vi "Instrument Meas CCDF (LTE).vi"(6 "Count(Kpt)":i32(ring) items=["0"=0, "1"=1, "10"=10, "100"=100, "1000"=1000, "10000"=10000], 7 "OPC?(T)":bool=TRUE, 8 "error in":errorcluster {"code" format="%.0x"}, 10 "Timeout":u32=10000, 11 "Session In":refnum<visa-resource-name>="GPIB0::18::INSTR") -> (0 "error out":errorcluster {"code" format="%.0x"}, 1 "Formatted Data":dbl[](array[numeric]), 2 "Data(str)":string[](array[string]), 3 "Session Out":refnum<visa-resource-name>)   [LabVIEW 2018]
doc: "Launches the Instrument I/O Assistant, which you can use to communicate with message-based instruments and graphically parse the response. For example you can communicate with an instrument that uses a serial, Ethernet, or GPIB interface."
panel:
  # "Returns 10 scalar results:\n0. Average input power (in dBm)\n1. Probability at the average input power level (in %)\n2. Power level that has 10% of the power\n3. Power level that has 1% of the power\n4. Power level that has 0.1% of the power\n5. Power level that has 0.01% of the power\n6. Power level that has 0.001% of the power\n7. Power level that has 0.0001% of the power\n8. Peak power (in dB)\n9.Count"
  # "Returns 10 scalar results:\n0. Average input power (in dBm)\n1. Peak  (in dB)\n2. Pk @ (dBm)"
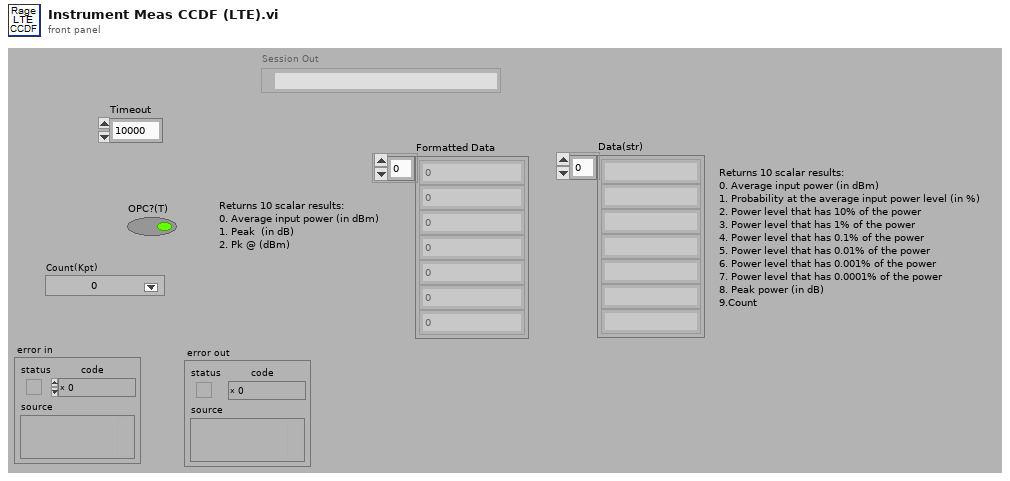
[diagram p1: front panel]
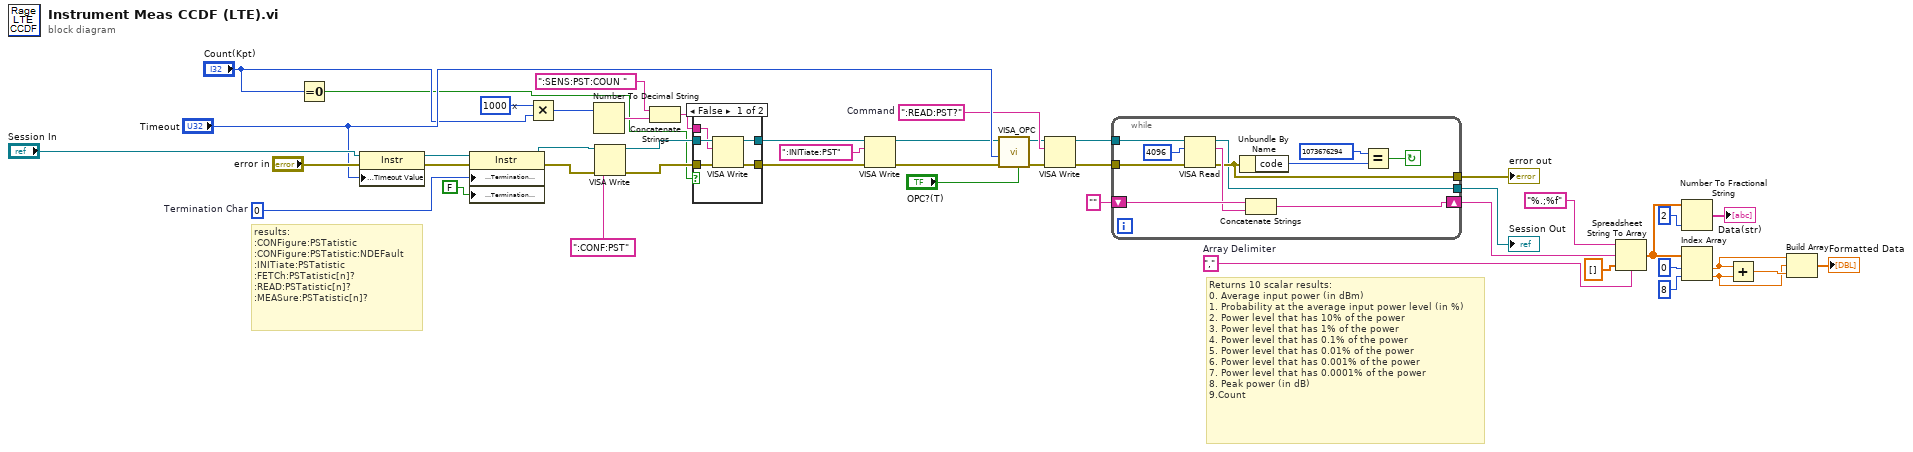
[diagram p0: block diagram]
diagram:
  w16 = ","  # Array Delimiter
  w19 = ":READ:PST?"  # Command
  w28 = 1000  # x
  w42 = u8 0  # Termination Char
  # "Returns 10 scalar results:\n0. Average input power (in dBm)\n1. Probability at the average input power level (in %)\n2. Power level that has 10% of the power\n3. Power level that has 1% of the power\n4. Power level that has 0.1% of the power\n5. Power level that has 0.01% of the power\n6. Power level that has 0.001% of the power\n7. Power level that has 0.0001% of the power\n8. Peak power (in dB)\n9.Count"
  # "results:\n:CONFigure:PSTatistic\n:CONFigure:PSTatistic:NDEFault\n:INITiate:PSTatistic\n:FETCh:PSTatistic[n]?\n:READ:PSTatistic[n]?\n:MEASure:PSTatistic[n]?"
  n1 = Equal To 0?(x="Count(Kpt)") -> (x = 0?=w26:bool)
  n2 = property class="Instr"(reference="Session In", error in="error in", "General Settings:Timeout Value"="Timeout") -> (reference out=w41:refnum<visa-resource-name>, error out=w44:errorcluster)
  n3 = property class="Instr"(reference=w41, error in=w44, "Message Based Settings:Termination Character"=w42, "Message Based Settings:Termination Character Enable"=FALSE ("enable")) -> (reference out=w38:refnum<visa-resource-name>, error out=w43:errorcluster)
  n4 = Multiply(x=w28, y="Count(Kpt)") -> (x*y=w29:i32)
  n5 = Number To Decimal String(number=w29) -> (decimal integer string=w32:string)  [unwired: 1 out]
  n6 = VISA Write(VISA resource name=w38, write buffer=":CONF:PST", error in (no error)=w43) -> (VISA resource name out=w34:refnum<visa-resource-name>, error out=w35:errorcluster)  [unwired: 1 out]
  n7 = Concatenate Strings(":SENS:PST:COUN " ("staticText"), w32) -> (w30:string)
  n8 = case shown="False" w26 {
    tunnel: [w51 w53] -> w36
    tunnel: w35 -> [w50 w53]
    tunnel: w34 -> [w49 w52]
    tunnel: [w48 w52] -> w33
    tunnel: w30 -> [w47 _]
    frame False {
      n9 = VISA Write(VISA resource name=w49, write buffer=w47, error in (no error)=w50) -> (VISA resource name out=w48:refnum<visa-resource-name>, error out=w51:errorcluster)  [unwired: 1 out]
    }
    frame True {
    }
  }
  n10 = VISA Write(VISA resource name=w33, write buffer=":INITiate:PST" ("StaticText"), error in (no error)=w36) -> (VISA resource name out=w13:refnum<visa-resource-name>, error out=w25:errorcluster)  [unwired: 1 out]
  n11 = call "VISA_OPC.vi"("OPC(T)"="OPC?(T)", "error in"=w25, "Timeout"="Timeout", "Session In"=w13) -> ("error out"=w14:errorcluster, "Session Out"=w9:refnum<visa-resource-name>)  [unwired: 5 in, 1 out]
  n12 = VISA Write(VISA resource name=w9, write buffer=w19, error in (no error)=w14) -> (VISA resource name out=w23:refnum<visa-resource-name>, error out=w22:errorcluster)  [unwired: 1 out]
  n13 = while {
    tunnel: w23 -> [w61]
    shift-right: [w55] -> w15
    shift-left: "" -> [w60]
    tunnel: w22 -> [w58]
    tunnel: [w57] -> w21
    tunnel: [w54] -> w2
    stop <- w56 continue-if-true
    n14 = VISA Read(VISA resource name=w61, byte count=u32 4096 ("byte count (0)"), error in (no error)=w58) -> (VISA resource name out=w54:refnum<visa-resource-name>, read buffer=w59:string, error out=w57:errorcluster)  [unwired: 1 out]
    n15 = Unbundle By Name(w57) -> ("code"=w63:i32)
    n16 = Concatenate Strings(w60, w59) -> (w55:string)
    n17 = Equal?(x=1073676294, y=w63) -> (x = y?=w56:bool)
  }
  "error out" <- w21
  "Session Out" <- w2
  n18 = Spreadsheet String To Array(delimiter (Tab)=w16, format string="%.;%f", spreadsheet string=w15, array type (2D Dbl)=dbl[] []) -> (array=w1:dbl[])
  n19 = Number To Fractional String(number=w1, precision (6)=i16 2) -> (F-format string=→"Data(str)":string[])  [unwired: 2 in]
  n20 = Index Array(array=w1, index #1=0 ("index"), index #2=8 ("index")) -> (element #1=w3:dbl, element #2=w4:dbl)
  n21 = Add(x=w3, y=w4) -> (x+y=w7:dbl)
  n22 = Build Array(w3, w4, w7) -> (→"Formatted Data":dbl[])
